vi "exeCLI.vi"(0 "Tab Control":T1(tab)=enum."Executable command line utilities", 5 "command line (interactive)":string="notepad LabVIEW.ini", 7 "command line (built-in)":string="cmd /c path", 9 "command line (utility)":string="sort /r", 11 "standard input":string="cat\nmouse\ndog") -> (4 "standard output":string, 6 "standard error":string, 8 "return code":i32)   [LabVIEW 2018]
doc: "You can use the System Exec VI to call command line utilities that return standard output to the command shell. You also can call interactive applications that you intend to launch using System Exec, but interact with using the UI of the executable."
panel:
  # "Overview: Demonstrates different ways to use the System Exec VI to programmatically run and pass parameters to interactive applications, built-in command line utilities, and executable command line utilities.\nRequirements: Windows\nInstructions:\n1. Select a System Exec VI use case by selecting one of the tabs of the tab control.\n2. Run the VI.\n3. View the results in the standard output window or in the application that opens."
  # "This case calls interactive applications that you intend to launch using System Exec, but interact with using the UI of the executable. In this case, you would not want to wait until completion and you would not want to run the application minimized. When calling such executables as notepad or mspaint, you need not enter the full path for the executable. These executables are found in the directories specified by the path environment variable for the command shell.  When calling executables not found in the directories specified by the path environment variable, you must include the full path to the executable in the command line.  If you are specifying a file as an input parameter, you may specifying the working directory to avoid passing the full path to the file in the command line.  In this case, the working directory was specified to point to the directory containing LabVIEW.ini."
  # "Use System Exec to call command line utilities that return standard output to the command shell. In this case, you would  want to wait until completion and run the application minimized. There are two types of command line utilities. The first type, shown below, are utilities built into the command shell, for example dir, del, path, etc. To run such commands, you must preface the command with \"cmd /c\". This calls cmd.exe, the command shell executable, and then calls the built-in command that you specify followed by any input parameters. Some commands also take standard input.  For an example that takes both input parameters and standard input, see the Executable command line utilities case."
  # "Use System Exec to call command line utilities that return standard output to the command shell. In this case, you would  want to wait until completion and run the application minimized. There are two types of command line utilities. The second type, shown below, are actually executables, for example sort, ipconfig, etc. To run such commands, specify the utility in the command line followed by any input parameters. In this case \"/r\" is used to specify a reverse sort. Some commands also take standard input. The \"sort\" command shown below takes \"cat\", \"mouse\", and \"dog\", sorts them alphabetically in reverse order, and returns the sorted list to standard output."
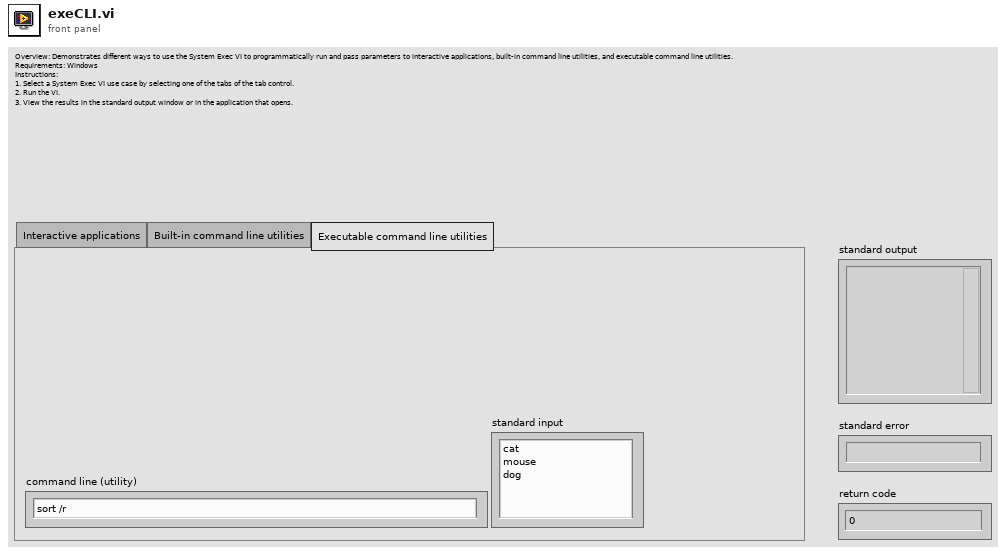
[diagram p1: front panel]
types:
  T1 = enum32{"Interactive applications", "Built-in command line utilities", "Executable command line utilities"}
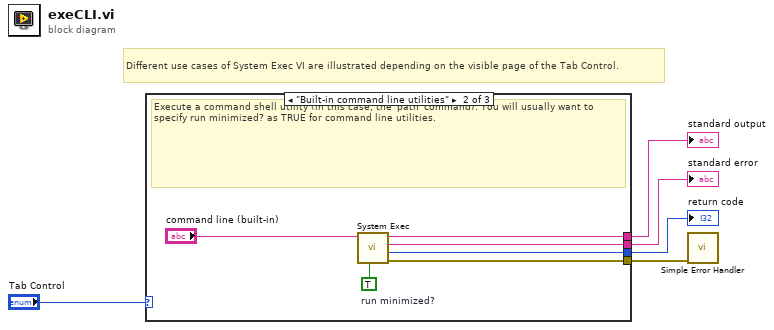
[diagram p0: block diagram]
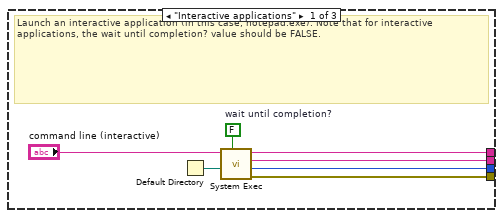
[diagram p2: hidden frame]
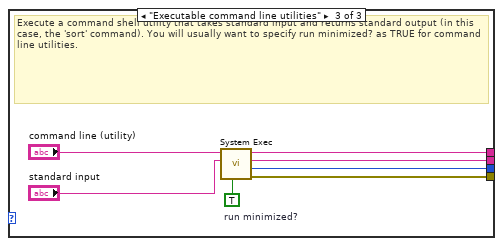
[diagram p3: hidden frame]
diagram:
  # "Different use cases of System Exec VI are illustrated depending on the visible page of the Tab Control."
  n1 = case shown="\"Built-in command line utilities\"" "Tab Control" {
    tunnel: [w9 w13 w20] -> w2
    tunnel: [w8 w14 w21] -> w5
    tunnel: [w7 w15 w22] -> w4
    tunnel: [w6 w16 w23] -> w3
    frame "Interactive applications" {
      w10 = FALSE  # wait until completion?
      # "Launch an interactive application (in this case, notepad.exe). Note that for interactive applications, the wait until completion? value should be FALSE."
      n2 = Default Directory() -> (w11:path)
      n3 = call <vilib>:"System Exec.vi"("wait until completion? (T)"=w10, "working directory"=w11, "command line"="command line (interactive)") -> ("error out"=w9:errorcluster, "return code"=w8:i32, "standard error"=w7:string, "standard output"=w6:string)  [unwired: 3 in, 2 out]
    }
    frame "Built-in command line utilities" {
      w17 = TRUE  # run minimized?
      # "Execute a command shell utility (in this case, the 'path' command). You will usually want to specify run minimized? as TRUE for command line utilities."
      n4 = call <vilib>:"System Exec.vi"("run minimized? (F)"=w17, "command line"="command line (built-in)") -> ("error out"=w13:errorcluster, "return code"=w14:i32, "standard error"=w15:string, "standard output"=w16:string)  [unwired: 4 in, 2 out]
    }
    frame "Executable command line utilities" {
      w24 = TRUE  # run minimized?
      # "Execute a command shell utility that takes standard input and returns standard output (in this case, the 'sort' command). You will usually want to specify run minimized? as TRUE for command line utilities."
      n5 = call <vilib>:"System Exec.vi"("run minimized? (F)"=w24, "standard input"="standard input", "command line"="command line (utility)") -> ("error out"=w20:errorcluster, "return code"=w21:i32, "standard error"=w22:string, "standard output"=w23:string)  [unwired: 3 in, 2 out]
    }
  }
  "return code" <- w5
  "standard error" <- w4
  "standard output" <- w3
  n6 = call <vilib>:"Simple Error Handler.vi"("error in (no error)"=w2) -> ()  [unwired: 1 in, 8 out]
